vi "Remove Unused Connections.vi"(11 "TCP Slave in":refnum<class "TCP Slave.lvclass">) -> (0 "error out":errorcluster)   [LabVIEW 2013, in "Modbus Library - Advance.lvlib" / "TCP Slave.lvclass"]
uses:
  TCP Slave.lvclass
  TCP Slave.lvclass/TCP Slave.ctl
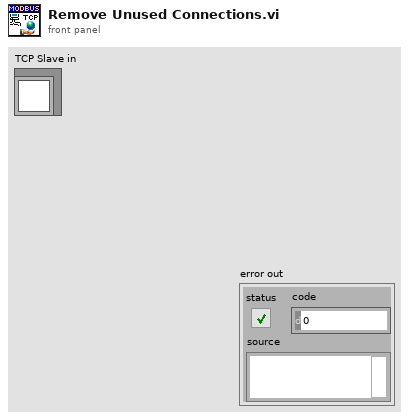
[diagram p1: front panel]
types:
  T1 = typedef "K2Labs Modbus Library.lvlib/TCP Slave.lvclass/Connection Counter.ctl" = cluster{"Currently Connected":u32, "Connection Records":refnum<data-value>[]}
  T2 = typedef "K2Labs Modbus Library.lvlib/TCP Slave.lvclass/Connection.ctl" = cluster{"Connected?":bool, "IP address":string, "Port":u16, "connection error":errorcluster}
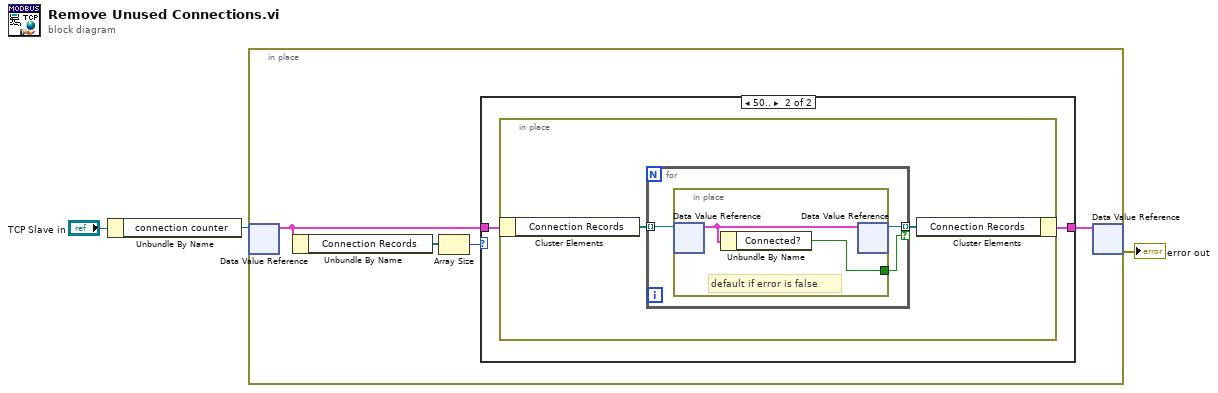
[diagram p0: block diagram]
diagram:
  n1 = Unbundle By Name("TCP Slave in") -> ("connection counter"=w1:refnum<data-value>)
  n2 = in-place {
    n3 = in-place-dvr #1(w1) -> (w4:T1)  [unwired: 1 out]
    n4 = Unbundle By Name(w4) -> ("Connection Records"=w6:refnum<data-value>[])
    n5 = Array Size(array=w6) -> (size(s)=w7:i32)
    n6 = case shown="50.." w7 {
      tunnel: [w8 w9] -> w5
      tunnel: w4 -> [w8 w10]
      frame Default {
      }
      frame 50.. {
        n7 = in-place {
          n8 = in-place-cluster #2(w10) -> ("Connection Records"=w12:refnum<data-value>[])
          n9 = for {
            tunnel: w12 -> [w15] mode=indexing
            tunnel: [w14] -> w11 mode=indexing if=w13
            n10 = in-place {
              in-place-border: [w16] -> w13
              # "default if error is false"
              n11 = in-place-dvr #3(w15) -> (w17:T2)  [unwired: 1 out]
              n12 = Unbundle By Name(w17) -> ("Connected?"=w16:bool)
              n13 = in-place-dvr #3(w17) -> (w14:refnum<data-value>)  [unwired: 1 out]
            }
          }
          n14 = in-place-cluster #2("Connection Records"=w11) -> (w9:T1)
        }
      }
    }
    n15 = in-place-dvr #1(w5) -> (→"error out":errorcluster)  [unwired: 1 out]
  }
